vi "sendTelMultiple.vi"(8 "error in (no error)":errorcluster, 9 "queueOptions":T2={"EnqueueOptions"=enum."normal enqueue", "Timeout (ms)"=0}, 10 "telemetry":T1[](array[typedef]), 11 "TcpServer in":refnum<class "TcpServer.lvclass">) -> (0 "error out":errorcluster, 2 "string":string, 3 "TcpServer out":refnum<class "TcpServer.lvclass">)   [LabVIEW 2018, in "TcpServer.lvclass"]
doc: "Send multiple telemetry to TCP Client. Use the queueOptions control to select lossy enqueue or normal enqueue, and timeout in ms.\n\nNote: this function will not handle any error internally, so the user must handle the errors when call it."
uses:
  TcpServer.lvclass
  TcpServerTel/typedef/queueOptionsTypeDef.ctl
  TcpServerTel/typedef/enqueueOptionsTypeDef.ctl
  TcpServerTel/typedef/telTypeDef.ctl
  TcpServer.lvclass/TcpServer.ctl
  TcpServerBase/typedef/msgTypeDef.ctl
  TcpServerTel/TcpServerTel.lvclass
  home/ttsai/Documents/github/ts_labview_tcp_json/src/TcpServerBase/TcpServerBase.lvclass
  TcpServerBase/TcpServerBase.lvclass
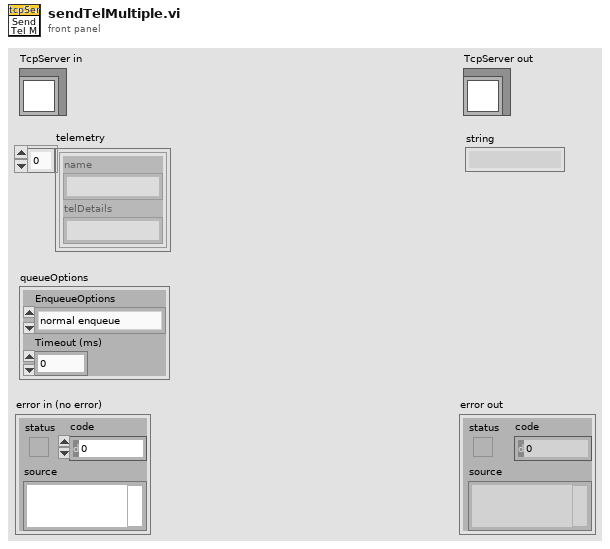
[diagram p1: front panel]
types:
  T1 = typedef "TcpServerTel.lvclass/telTypeDef.ctl" = cluster{"name":string, "telDetails":string}
  T2 = typedef "TcpServerTel.lvclass/queueOptionsTypeDef.ctl" = cluster{"EnqueueOptions":T3, "Timeout (ms)":i32}
  T3 = typedef "TcpServerTel.lvclass/enqueueOptionsTypeDef.ctl" = enum16{"lossy enqueue", "normal enqueue"}
  T4 = typedef "TcpServerBase.lvclass/msgTypeDef.ctl" = cluster{"msgName":string, "msgDetails":string}
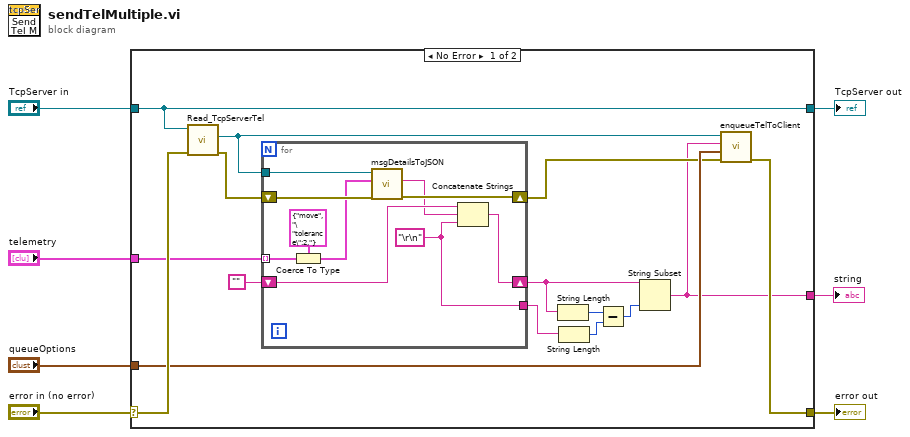
[diagram p0: block diagram]
diagram:
  n1 = case shown="No Error" "error in (no error)" {
    selector: "error in (no error)" -> [w21 w34]
    tunnel: [w9 w34] -> w6
    tunnel: [w22 w33] -> w4
    tunnel: "TcpServer in" -> [w22 w33]
    tunnel: "telemetry" -> [w20 _]
    tunnel: "queueOptions" -> [w11 _]
    tunnel: [w8 _] -> w1
    frame No Error {
      n2 = call "Read_TcpServerTel.vi"("error in (no error)"=w21, "TcpServer in"=w22) -> ("error out"=w19:errorcluster, "TcpServerTel.lvclass"=w12:refnum<class "TcpServerTel.lvclass">)  [unwired: 7 in, 1 out]
      n3 = for {
        tunnel: w20 -> [w31] mode=indexing
        tunnel: w12 -> [w30]
        shift-right: [w27] -> w10
        shift-left: w19 -> [w29]
        shift-right: [w24] -> w16
        shift-left: "" -> [w26]
        tunnel: [w23] -> w17
        w23 = "\r\n" ("string")
        n4 = Coerce To Type(0:w31, 1:T4 {"msgName"="move", "msgDetails"="\"tolerance\":2,"} ("msgData")) -> (2:w28:T4)
        n5 = call "msgDetailsToJSON.vi"("error in (no error)"=w29, "msgData"=w28, "TcpServerBase in"=w30) -> ("error out"=w27:errorcluster, "JSON string"=w25:string)  [unwired: 6 in, 1 out]
        n6 = Concatenate Strings(w26, w25, w23) -> (w24:string)
      }
      n7 = String Length(string=w16) -> (length=w15:i32)
      n8 = String Length(string=w17) -> (length=w14:i32)
      n9 = Subtract(x=w15, y=w14) -> (x-y=w13:i32)
      n10 = String Subset(string=w16, length (rest)=w13) -> (substring=w8:string)  [unwired: 1 in]
      n11 = call "enqueueTelToClient.vi"("error in (no error)"=w10, "queueOptions"=w11, "elements to enqueue"=w8, "TcpServerTel in"=w12) -> ("error out"=w9:errorcluster)  [unwired: 6 in, 1 out]
    }
    frame Error {
    }
  }
  "error out" <- w6
  "TcpServer out" <- w4
  "string" <- w1
